vi "Remove Path.vi"(11 "Include Paths Ref":refnum<vi> caption="包括路径引用") -> (1 "Path Strings Out":T1 caption="路径字符串输出", 3 "Dup Include Paths Ref":refnum<vi> caption="包括路径引用副本")   [LabVIEW 2011, in "NISAST Include Paths.xctl"]
uses:
  NISAST Include Paths.xctl
  Data.ctl
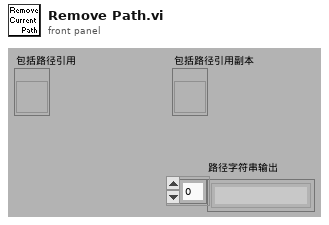
[diagram p1: front panel]
types:
  T1 = typedef "NISAST Include Paths.xctl/Data.ctl" = string[]
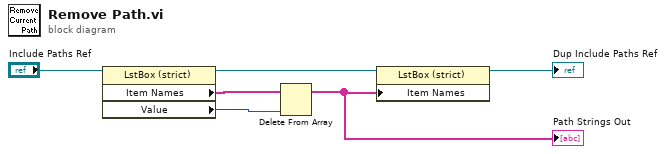
[diagram p0: block diagram]
diagram:
  n1 = property class="LstBox (strict)"(reference="Include Paths Ref") -> (reference out=w6:refnum<vi>, "Item Names"=w3:string[], "Value"=w2:i32)  [unwired: 1 in, 1 out]
  n2 = Delete From Array(array=w3, index=w2) -> (array with subset deleted=w1:string[])  [unwired: 1 in, 1 out]
  "Path Strings Out" <- w1
  n3 = property class="LstBox (strict)"(reference=w6, "Item Names"=w1) -> (reference out=→"Dup Include Paths Ref":refnum<vi>)  [unwired: 1 in, 1 out]
